vi "DMM_Frequency Domain Meas Format Function Range.vi"(0 "DMM Handle In":refnum<k15>, 5 "Function Settings In":T4={"Resolution in Digits"=5.5, "Range and Function"=enum."Frequency AC Auto Range"} {"Resolution in Digits" items=["3 1/2"=3.5, "4 1/2"=4.5, "5 1/2"=5.5, "6 1/2"=6.5, "7 1/2"=7.5]}, 11 "error in":errorcluster) -> (4 "DMM Handle Out":refnum<k15>, 6 "Function Settings Out":T3={"Frequency Range"=0.0, "Function"=enum."DC Volts", "Vertical Range"=0.0, "Resolution in Digits"=5.5} {"Resolution in Digits" items=["3 1/2"=3.5, "4 1/2"=4.5, "5 1/2"=5.5, "6 1/2"=6.5, "7 1/2"=7.5]}, 15 "error out":errorcluster)   [LabVIEW 2021, in "DMM_Frequency Domain Measurement.lvlib"]
doc: "Utilizes the function settings input to select the particular function and range used for the measurement and format the output string displayed in the measurement output cluster."
uses:
  DMM_Frequency Domain Measurement.lvlib
  Typedefs/Function Settings.ctl
  <instrlib>/niDMM/nidmm.llb/niDMM Resolution in Digits.ctl
  <instrlib>/niDMM/nidmm.llb/niDMM Function.ctl
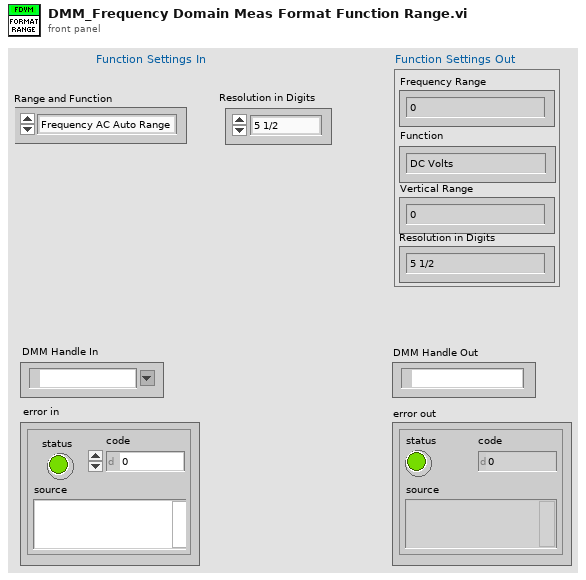
[diagram p1: front panel]
types:
  T1 = typedef "niDMM Function.ctl" = enum16{"DC Volts", "AC Volts", "DC Current", "AC Current", "2-wire Resistance", "4-wire Resistance", "Diode", "Frequency", "Period", "AC Volts DC Coupled", "Capacitance", "Inductance", "Temperature"}
  T2 = typedef "niDMM Resolution in Digits.ctl" = dbl
  T3 = cluster{"Frequency Range":dbl, "Function":T1, "Vertical Range":dbl, "Resolution in Digits":T2}
  T4 = typedef "DMM_Frequency Domain Measurement.lvlib/Function Settings.ctl" = cluster{"Resolution in Digits":T2, "Range and Function":enum16{"Frequency AC Auto Range", "Freq AC 50 mV", "Freq AC 500 mV", "Freq AC 5 V", "Freq AC 50 V", "Freq AC 300 V", "      ", "Period AC Auto Range", "Period AC 50 mV", "Period AC 500 mV", "Period AC 5 V", "Period AC 50 V", "Period AC 300 V"}}
  T5 = cluster{"Range":dbl, "Function":T1, "Freq_Period AC Range":dbl, "Resolution in Digits":T2}
  T6 = enum16{"Frequency AC Auto Range", "Freq AC 50 mV", "Freq AC 500 mV", "Freq AC 5 V", "Freq AC 50 V", "Freq AC 300 V", "      ", "Period AC Auto Range", "Period AC 50 mV", "Period AC 500 mV", "Period AC 5 V", "Period AC 50 V", "Period AC 300 V"}
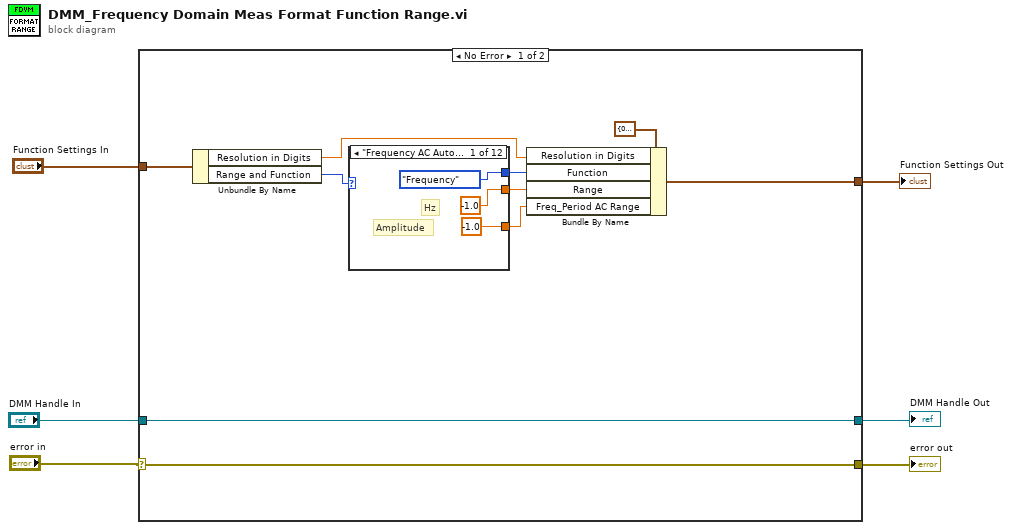
[diagram p0: block diagram]
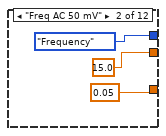
[diagram p2: hidden frame]
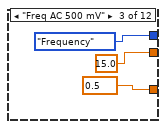
[diagram p3: hidden frame]
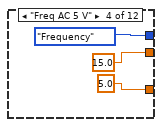
[diagram p4: hidden frame]
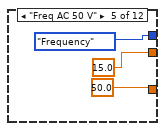
[diagram p5: hidden frame]
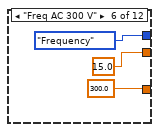
[diagram p6: hidden frame]
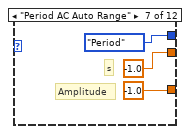
[diagram p7: hidden frame]
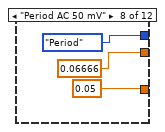
[diagram p8: hidden frame]
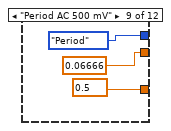
[diagram p9: hidden frame]
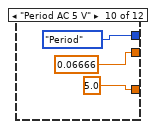
[diagram p10: hidden frame]
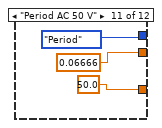
[diagram p11: hidden frame]
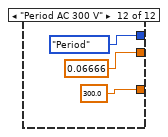
[diagram p12: hidden frame]
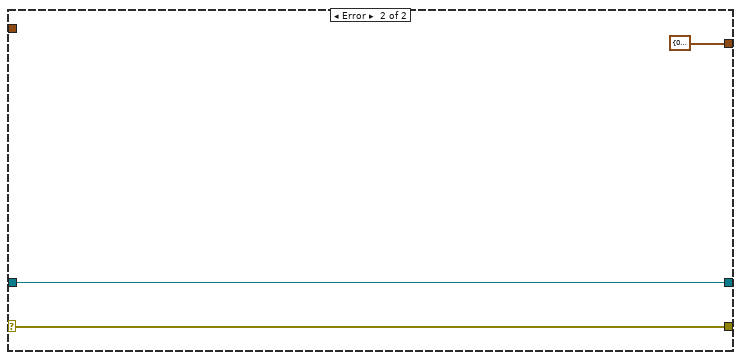
[diagram p13: hidden frame]
diagram:
  n1 = case shown="No Error" "error in" {
    selector: "error in" -> [w14 w54]
    tunnel: "Function Settings In" -> [w16 _]
    tunnel: [w11 T5 {"Range"=0.0, "Function"=enum."DC Volts", "Freq_Period AC Range"=0.0, "Resolution in Digits"=5.5} ("Function Settings Out")] -> w1
    tunnel: [w14 w54] -> w5
    tunnel: [w13 w55] -> w3
    tunnel: "DMM Handle In" -> [w13 w55]
    frame No Error {
      n2 = Unbundle By Name(w16) -> ("Resolution in Digits"=w15:T2, "Range and Function"=w10:T6)
      n3 = case shown="\"Frequency AC Auto Range\", Default" w10 {
        tunnel: [niDMM_Function."Frequency" ("Function") niDMM_Function."Frequency" ("Function") niDMM_Function."Frequency" ("Function") niDMM_Function."Frequency" ("Function") niDMM_Function."Frequency" ("Function") niDMM_Function."Frequency" ("Function") niDMM_Function."Period" ("Function") niDMM_Function."Period" ("Function") niDMM_Function."Period" ("Function") niDMM_Function."Period" ("Function") niDMM_Function."Period" ("Function") niDMM_Function."Period" ("Function")] -> w9
        tunnel: [-1.0 ("Range") 15.0 ("Range") 15.0 ("Range") 15.0 ("Range") 15.0 ("Range") 15.0 ("Range") -1.0 ("Range") 0.06666 ("Range") 0.06666 ("Range") 0.06666 ("Range") 0.06666 ("Range") 0.06666 ("Range")] -> w8
        tunnel: [-1.0 ("Range") 0.05 ("Range") 0.5 ("Range") 5.0 ("Range") 50.0 ("Range") 300.0 ("Range") -1.0 ("Range") 0.05 ("Range") 0.5 ("Range") 5.0 ("Range") 50.0 ("Range") 300.0 ("Range")] -> w7
        frame "Frequency AC Auto Range", Default {
          # "Amplitude"
          # "Hz"
        }
        frame "Freq AC 50 mV" {
        }
        frame "Freq AC 500 mV" {
        }
        frame "Freq AC 5 V" {
        }
        frame "Freq AC 50 V" {
        }
        frame "Freq AC 300 V" {
        }
        frame "Period AC Auto Range" {
          # "Amplitude"
          # "s"
        }
        frame "Period AC 50 mV" {
        }
        frame "Period AC 500 mV" {
        }
        frame "Period AC 5 V" {
        }
        frame "Period AC 50 V" {
        }
        frame "Period AC 300 V" {
        }
      }
      n4 = Bundle By Name(cluster=T5 {"Range"=0.0, "Function"=enum."DC Volts", "Freq_Period AC Range"=0.0, "Resolution in Digits"=5.5} ("Function Settings Out"), "Resolution in Digits"=w15, "Function"=w9, "Range"=w8, "Freq_Period AC Range"=w7) -> (w11:T5)
    }
    frame Error {
    }
  }
  "error out" <- w5
  "DMM Handle Out" <- w3
  "Function Settings Out" <- w1
